vi "More Dialog.vi"(11 "FGEN Sample Rate (Reference)":dbl format="%#_6pHz") -> ()   [LabVIEW 2025, in "FGEN Arb Sequence Mode UI.lvlib"]
doc: "Use this template to build a producer/consumer design pattern with events to produce queue items. Use this design pattern instead of the User Interface Event Handler pattern for user interfaces when you want to execute code asynchronously in response to an event without slowing the user interface responsiveness."
uses:
  FGEN Arb Sequence Mode UI.lvlib
panel:
  in  "Calculate Marker Position and Copy":bool
  in  "FGEN Sample Rate (For Calc)":dbl caption="FGEN Sample Rate" format="%#_6pHz"
  out "Marker Postion":i32
  in  "Time in Seconds":dbl format="%#_6ps"
  # "Marker Position Calculator"
  # "="
  # "X"
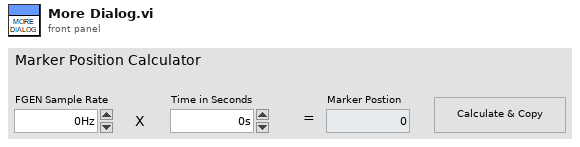
[diagram p1: front panel]
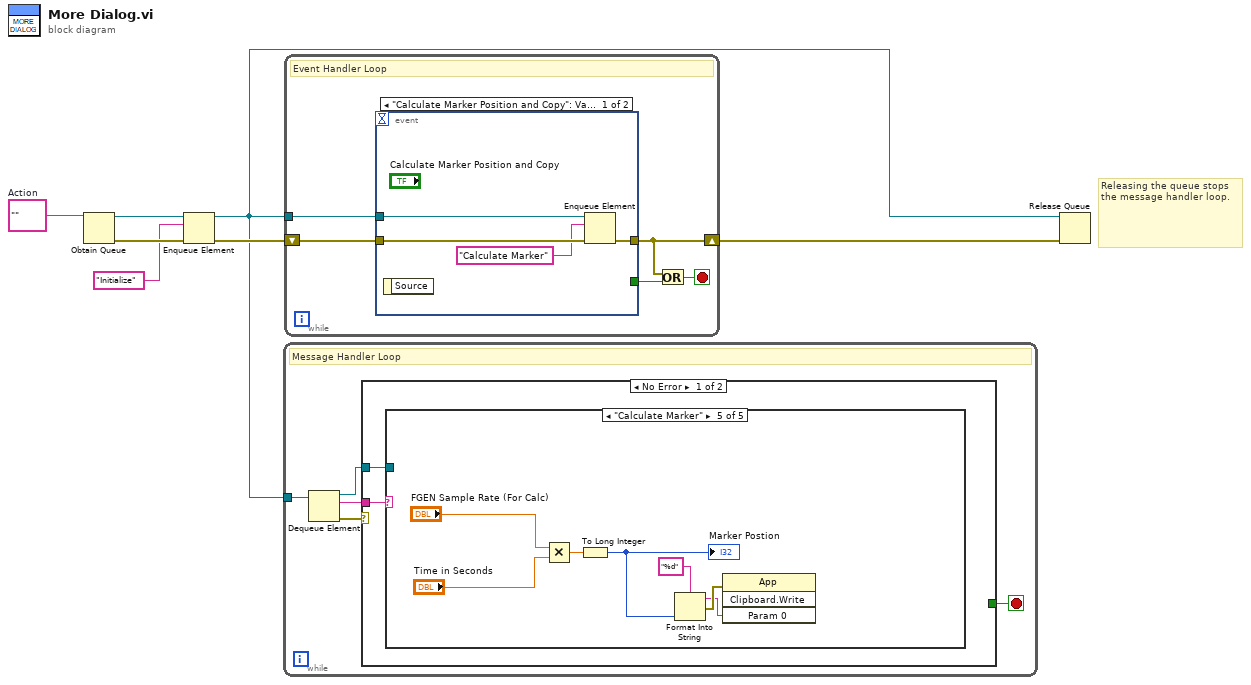
[diagram p0: block diagram]
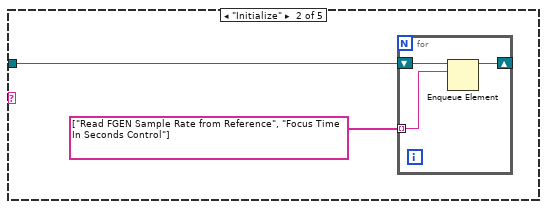
[diagram p3: hidden frame]
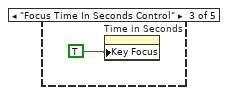
[diagram p4: hidden frame]
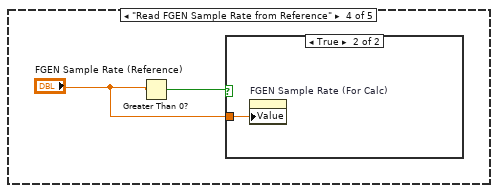
[diagram p5: hidden frame]
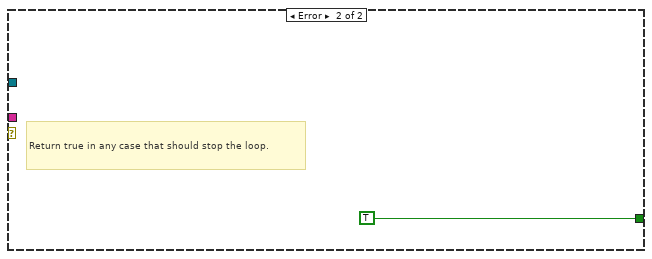
[diagram p7: hidden frame]
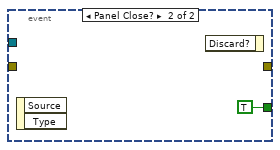
[diagram p8: hidden frame]
diagram:
  w5 = ""  # Action
  # "Releasing the queue stops the message handler loop."
  n1 = Obtain Queue(element data type=w5) -> (queue out=w3:refnum<queue>, error out=w7:errorcluster)  [unwired: 4 in, 1 out]
  n2 = Enqueue Element(queue=w3, element="Initialize", error in (no error)=w7) -> (queue out=w2:refnum<queue>, error out=w4:errorcluster)  [unwired: 1 in, 1 out]
  n3 = while {
    tunnel: w2 -> [w12]
    stop <- w9 stop-if-true
    # "Message Handler Loop"
    n4 = Dequeue Element(queue=w12) -> (queue out=w8:refnum<queue>, element=w10:string, error out=w11:errorcluster)  [unwired: 2 in, 1 out]
    n5 = case shown="No Error" w11 {
      tunnel: w10 -> [w14 _]
      tunnel: [_ TRUE] -> w9
      tunnel: w8 -> [w13 _]
      frame No Error {
        n6 = case shown="\"Calculate Marker\"" w14 {
          tunnel: w13 -> [_ w15 _ _ _]
          frame Default {
          }
          frame "Initialize" {
            n7 = for {
              tunnel: string[] ["Read FGEN Sample Rate from Reference", "Focus Time In Seconds Control"] ("element") -> [w19] mode=indexing
              shift-right: [w17] -> _
              shift-left: w15 -> [w18]
              n8 = Enqueue Element(queue=w18, element=w19) -> (queue out=w17:refnum<queue>)  [unwired: 2 in, 2 out]
            }
          }
          frame "Focus Time In Seconds Control" {
            n9 = property on="Time in Seconds" class="DigNum (strict)"("Key Focus"=TRUE) -> ()  [unwired: 2 in, 2 out]
          }
          frame "Read FGEN Sample Rate from Reference" {
            n10 = Greater Than 0?(x="FGEN Sample Rate (Reference)") -> (x > 0?=w22:bool)
            n11 = case shown="True" w22 {
              tunnel: "FGEN Sample Rate (Reference)" -> [_ w23]
              frame False {
              }
              frame True {
                n12 = property on="FGEN Sample Rate (For Calc)" class="DigNum (strict)"("Value"=w23) -> ()  [unwired: 2 in, 2 out]
              }
            }
          }
          frame "Calculate Marker" {
            n13 = Multiply(x="FGEN Sample Rate (For Calc)", y="Time in Seconds") -> (x*y=w27:dbl)
            n14 = To Long Integer(number=w27) -> (32bit integer=w24:i32)
            "Marker Postion" <- w24
            n15 = Format Into String(format string="%d", w24) -> (resulting string=w26:string, error out=w28:errorcluster)  [unwired: 2 in]
            n16 = invoke class="App" method="Clipboard.Write"(error in=w28, "Param 0"=w26) -> ()  [unwired: 2 in, 4 out]
          }
        }
      }
      frame Error {
        # "Return true in any case that should stop the loop."
      }
    }
  }
  n17 = while {
    shift-right: [w32] -> w6
    shift-left: w4 -> [w35]
    tunnel: w2 -> [w36]
    stop <- w33 stop-if-true
    # "Event Handler Loop"
    n18 = event shown="[0] \"Calculate Marker Position and Copy\": Value Change" {
      selector: _ -> [_ _]
      dyn-events: _ -> [_ _]
      timeout: _ -> [_ _]
      tunnel: w36 -> [w40 _]
      tunnel: w35 -> [w39 _]
      tunnel: [w38 _] -> w32
      tunnel: [_ TRUE ("stop")] -> w34
      event "Calculate Marker Position and Copy": Value Change {
        n19 = event-data() -> ()  [unwired: 1 in, 1 out]
        n20 = Enqueue Element(queue=w40, element="Calculate Marker", error in (no error)=w39) -> (error out=w38:errorcluster)  [unwired: 1 in, 2 out]
      }
      event Panel Close? {
        n21 = event-data() -> ()  [unwired: 1 in, 2 out]
        n22 = event-data() -> ()  [unwired: 2 in, 1 out]
      }
    }
    n23 = Or(x=w32, y=w34) -> (x .or. y?=w33:bool)
  }
  n24 = Release Queue(queue=w2, error in (no error)=w6) -> ()  [unwired: 1 in, 3 out]
